vi "Sweep2614_NoRecord.vi"(1 "Time step (sec)":dbl=0.1, 2 "Rate (V/min)":dbl=30.0, 3 "Vfinal (V)":dbl, 4 "GPIB":string="12") -> (0 "Vinitial (V)":dbl)   [LabVIEW 2017]
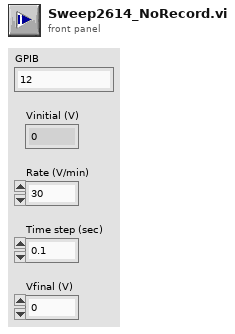
[diagram p1: front panel]
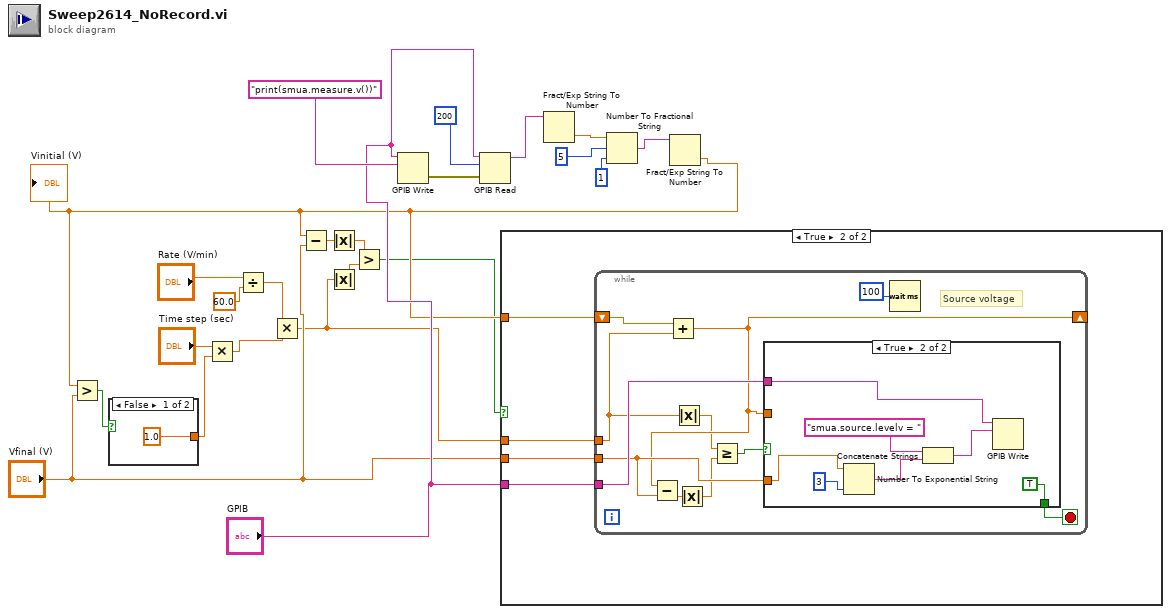
[diagram p0: block diagram]
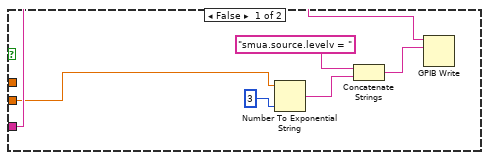
[diagram p2: hidden frame]
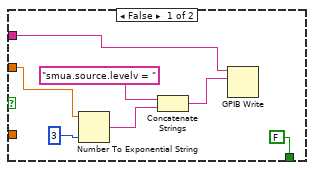
[diagram p3: hidden frame]
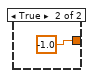
[diagram p4: hidden frame]
diagram:
  n1 = Divide(x="Rate (V/min)", y=60.0) -> (x/y=w23:dbl)
  n2 = GPIB Write(0:"GPIB", 1:"print(smua.measure.v())" ("data")) -> (6:w20:errorcluster)  [unwired: 3 in, 1 out]
  n3 = GPIB Read(0:"GPIB", 1:200 ("byte count"), 3:w20) -> (5:w9:string)  [unwired: 2 in, 2 out]
  n4 = Fract/Exp String To Number(string=w9) -> (number=w12:dbl)  [unwired: 3 in, 1 out]
  n5 = Number To Fractional String(number=w12, width (-)=5, precision (6)=1) -> (F-format string=w8:string)  [unwired: 1 in]
  n6 = Fract/Exp String To Number(string=w8) -> (number=w7:dbl)  [unwired: 3 in, 1 out]
  "Vinitial (V)" <- w7
  n7 = Greater?(x=w7, y="Vfinal (V)") -> (0:w16:bool)
  n8 = case shown="False" w16 {
    tunnel: [1.0 -1.0] -> w13
    frame False {
    }
    frame True {
    }
  }
  n9 = Multiply(x="Time step (sec)", y=w13) -> (x*y=w14:dbl)
  n10 = Multiply(x=w23, y=w14) -> (x*y=w4:dbl)
  n11 = Subtract(x=w7, y="Vfinal (V)") -> (x-y=w5:dbl)
  n12 = Absolute Value(x=w5) -> (abs(x)=w3:dbl)
  n13 = Absolute Value(x=w4) -> (abs(x)=w2:dbl)
  n14 = Greater?(x=w3, y=w2) -> (0:w1:bool)
  n15 = case shown="True" w1 {
    tunnel: w4 -> [_ w35]
    tunnel: "GPIB" -> [w27 w34]
    tunnel: "Vfinal (V)" -> [w26 w33]
    tunnel: w7 -> [_ w32]
    frame False {
      n16 = Number To Exponential String(number=w26, precision (6)=3) -> (E-format string=w30:string)  [unwired: 2 in]
      n17 = Concatenate Strings("smua.source.levelv = ", w30) -> (w29:string)
      n18 = GPIB Write(0:w27, 1:w29) -> ()  [unwired: 3 in, 2 out]
    }
    frame True {
      n19 = while {
        shift-right: [w40] -> _
        shift-left: w32 -> [w46]
        tunnel: w35 -> [w36]
        tunnel: w33 -> [w41]
        tunnel: w34 -> [w42]
        stop <- w44 stop-if-true
        # "Source voltage"
        n20 = Add(x=w46, y=w36) -> (x+y=w40:dbl)
        n21 = Subtract(x=w40, y=w41) -> (x-y=w39:dbl)
        n22 = Absolute Value(x=w36) -> (abs(x)=w37:dbl)
        n23 = Absolute Value(x=w39) -> (abs(x)=w38:dbl)
        n24 = Greater Or Equal?(x=w37, y=w38) -> (x >= y?=w45:bool)
        n25 = case shown="True" w45 {
          tunnel: w40 -> [w49 _]
          tunnel: w41 -> [_ w56]
          tunnel: w42 -> [w48 w55]
          tunnel: [FALSE TRUE] -> w44
          frame False {
            n26 = Number To Exponential String(number=w49, precision (6)=3) -> (E-format string=w52:string)  [unwired: 2 in]
            n27 = Concatenate Strings("smua.source.levelv = ", w52) -> (w51:string)
            n28 = GPIB Write(0:w48, 1:w51) -> ()  [unwired: 3 in, 2 out]
          }
          frame True {
            n29 = Number To Exponential String(number=w56, precision (6)=3) -> (E-format string=w59:string)  [unwired: 2 in]
            n30 = Concatenate Strings("smua.source.levelv = ", w59) -> (w58:string)
            n31 = GPIB Write(0:w55, 1:w58) -> ()  [unwired: 3 in, 2 out]
          }
        }
        n32 = Wait (ms)(milliseconds to wait=100) -> ()  [unwired: 1 out]
      }
    }
  }
